vi "HFRR ADV v018 new software.vi"() -> ()   [LabVIEW 2025] (continued)
              }
            }
          }
        }
        n4002 = disable-structure shown="Disabled" {
          disable-tunnel: w4768 -> [w4777 _]
          disable-tunnel: [w4776 _] -> w4767
          frame Disabled {
            n4003 = local read "Json St Flg"() -> (w4775:bool)
            n4004 = case shown="True" w4775 {
              tunnel: w4777 -> [w4778 w4780]
              tunnel: [w4778 w4779] -> w4776
              frame False {
              }
              frame True {
                n4005 = Increment(x=w4780) -> (x+1=w4779:dbl)
                "T cycle" <- w4779
                n4006 = local write "Json St Flg"(FALSE ("Json St Flg")) -> ()
              }
            }
          }
          frame Enabled {
          }
        }
        n4007 = local read "Quit"() -> (w4762:bool)
      }
    }
    frame Enabled {
    }
  }
  n4008 = stacked-sequence {
    tunnel: [w5160] -> w40
    frame #0 {
      w5160 = FALSE ("Upload \nConfirmed")
      n4009 = local write "Upload \nConfirmed"(w5160) -> ()
      n4010 = local write "St Str"("") -> ()
    }
  }
  n4011 = disable-structure shown="Disabled" {
    disable-tunnel: w40 -> [w5161 _]
    frame Disabled {
      n4012 = case shown="True" {
        selector: _ -> [_ _]
        tunnel: w5161 -> [_ w5162]
        frame False {
        }
        frame True {
          n4013 = while {
            tunnel: [w5168] -> _
            tunnel: w5162 -> [_]
            i -> [w5168]
            stop <- w5163 stop-if-true
            n4014 = local read "Json End Flg"() -> (w5167:bool)
            n4015 = Wait (ms)(milliseconds to wait=u32 20 ("Refresh Rate (ms)")) -> ()  [unwired: 1 out]
            n4016 = local read "refresh flag"() -> (w5164:bool)
            n4017 = local read "RUN"() -> (w5165:bool)
            n4018 = And(x=w5165, y=w5164) -> (x .and. y?=w5166:bool)
            n4019 = Or(x=w5166, y=w5167) -> (x .or. y?=w5169:bool)
            "AR Led" <- w5169
            n4020 = case shown="True" w5169 {
              frame False {
              }
              frame True {
                w5186 = "\",\""
                n4021 = local read "UUID"() -> (w5184:string)
                n4022 = local write "refresh flag"(FALSE ("refresh flag")) -> ()
                n4023 = local read "time"() -> (w5173:dbl)
                n4024 = Multiply(x=w5173, y=60.0) -> (x*y=w5172:dbl)
                n4025 = Concatenate Strings("UUID\" : \"", w5184, "\"}") -> (w5187:string)
                n4026 = Number To Fractional String(number=w5172, width (-)=i16 10, precision (6)=i16 4) -> (F-format string=w5201:string)  [unwired: 1 in]
                n4027 = Concatenate Strings("{", "\"Time\":\"", w5201, w5186) -> (w5196:string)
                n4028 = stacked-sequence {
                  tunnel: w5186 -> [w5249 w5257 w5264 w5272 w5280 w5289 w5296]
                  tunnel: [w5250 _ _ _ _ _ _] -> w5200
                  tunnel: [_ w5258 _ _ _ _ _] -> w5199
                  tunnel: [_ _ w5265 _ _ _ _] -> w5198
                  tunnel: [_ _ _ w5274 _ _ _] -> w5197
                  tunnel: w5187 -> [_ _ _ _ _ _ w5307]
                  tunnel: [_ _ _ _ _ _ w5306] -> w5183
                  tunnel: [_ _ _ _ _ w5286 _] -> w5182
                  tunnel: [_ _ _ _ w5279 _ _] -> w5181
                  frame #0 {
                    n4029 = local read "NORMAL LOAD"() -> (w5248:dbl)
                    n4030 = Number To Fractional String(number=w5248, width (-)=i16 10, precision (6)=i16 4) -> (F-format string=w5251:string)  [unwired: 1 in]
                    n4031 = Concatenate Strings("NormalLoad\":\"", w5251, w5249) -> (w5250:string)
                  }
                  frame #1 {
                    n4032 = local read "Temp"() -> (w5256:dbl)
                    n4033 = Number To Fractional String(number=w5256, width (-)=i16 10, precision (6)=i16 4) -> (F-format string=w5259:string)  [unwired: 1 in]
                    n4034 = Concatenate Strings("Temperature\":\"", w5259, w5257) -> (w5258:string)
                  }
                  frame #2 {
                    n4035 = local read "cof"() -> (w5262:dbl)
                    n4036 = Number To Fractional String(number=w5262, width (-)=i16 10, precision (6)=i16 4) -> (F-format string=w5266:string)  [unwired: 1 in]
                    n4037 = Concatenate Strings("FrictionalForce\":\"", w5266, w5264) -> (w5265:string)
                  }
                  frame #3 {
                    n4038 = local read "Set Hz"() -> (w5270:dbl)
                    n4039 = Multiply(x=w5270, y=60.0) -> (x*y=w5269:dbl)
                    n4040 = Number To Fractional String(number=w5269, width (-)=i16 10, precision (6)=i16 4) -> (F-format string=w5275:string)  [unwired: 1 in]
                    n4041 = Concatenate Strings("Speed\":\"", w5275, w5272) -> (w5274:string)
                  }
                  frame #4 {
                    n4042 = local read item#-1() -> (w5278)
                    n4043 = Number To Fractional String(number=w5278, width (-)=i16 10, precision (6)=i16 4) -> (F-format string=w5282:string)  [unwired: 1 in]
                    n4044 = Concatenate Strings("LinearDeformation\":\"", w5282, w5280) -> (w5279:string)
                  }
                  frame #5 {
                    n4045 = local read "AIR TEMP"() -> (w5285:dbl)
                    n4046 = local read "Json St Flg"() -> (w5287:bool)
                    n4047 = local read "Json End Flg"() -> (w5288:bool)
                    n4048 = Number To Fractional String(number=w5285, width (-)=i16 10, precision (6)=i16 4) -> (F-format string=w5291:string)  [unwired: 1 in]
                    n4049 = Concatenate Strings("Vibration\":\"", w5291, w5289) -> (w5286:string)
                    n4050 = And(x=w5287, y=w5288) -> ()  [unwired: 1 out]
                  }
                  frame #6 {
                    n4051 = local read "Json End Flg"() -> (w5295:bool)
                    n4052 = Get Date/Time In Seconds() -> (seconds since 1Jan1904=w5303:timestamp)
                    n4053 = local read "Json St Flg"() -> (w5294:bool)
                    n4054 = To Double Precision Float(number=w5303) -> (double precision float=w5302:dbl)
                    n4055 = Subtract(x=w5302, y=2082844800.0) -> (x-y=w5300:dbl)
                    n4056 = Number To Fractional String(number=w5300, width (-)=i16 12, precision (6)=i16 0) -> (F-format string=w5297:string)  [unwired: 1 in]
                    n4057 = case shown="True" w5295 {
                      tunnel: ["" w5310] -> w5304
                      tunnel: w5297 -> [_ w5311]
                      tunnel: w5296 -> [_ w5309]
                      frame False {
                      }
                      frame True {
                        n4058 = local write "Json End Flg"(FALSE ("Json St Flg")) -> ()
                        n4059 = Concatenate Strings("End\": \"", w5311, w5309) -> (w5310:string)
                      }
                    }
                    n4060 = case shown="True" w5294 {
                      tunnel: [w5314 w5317] -> w5305
                      tunnel: w5297 -> [_ w5318]
                      tunnel: w5296 -> [_ w5315]
                      frame False {
                        n4061 = local read "St Str"() -> (w5314:string)
                      }
                      frame True {
                        n4062 = Concatenate Strings("Start\":\"", w5318, w5315) -> (w5317:string)
                        "St Str" <- w5317
                        n4063 = local write "Json St Flg"(FALSE ("Json St Flg")) -> ()
                      }
                    }
                    n4064 = Concatenate Strings(w5305, w5304, w5307) -> (w5306:string)
                  }
                }
                n4065 = local read "FILE"() -> (w5175:string)
                n4066 = Concatenate Strings("\",\"OperatorID\":\"" ("string"), "Operator ID") -> (w5178:string)
                n4067 = Concatenate Strings("\",\"DatasetTitle\":\"" ("string"), w5175) -> (w5177:string)
                n4068 = Concatenate Strings("\",\"SerialNumber\":\"" ("string"), "Serial No") -> (w5207:string)
                n4069 = Concatenate Strings("\",\"ModelNumber\":\"" ("string"), "Model No") -> (w5206:string)
                n4070 = Concatenate Strings(w5207, w5206) -> (w5189:string)
                n4071 = Concatenate Strings("{\"SecretKey\":\"", "Secret Key", w5189, w5178, w5177, "\",\"Samples\":[") -> (w5194:string)
                n4072 = Concatenate Strings(w5196, w5200, w5199, w5198, w5197, w5181, w5182, w5183) -> (w5195:string)
                n4073 = Concatenate Strings(w5194, w5195, "]}") -> (w5193:string)
                n4074 = stacked-sequence {
                  tunnel: w5193 -> [w5222 _ _]
                  tunnel: [_ _ w5239] -> _
                  frame #0 {
                    (unwired) FALSE ("convert eol (F)")
                    w5224 = enum16{"start", "end", "current"}."start" ("pos mode (0:2)")
                    n4075 = Path To String(path="Path") -> (string=w5230:string)
                    n4076 = Concatenate Strings(w5230, "\\", "Data File Name") -> (w5232:string)
                    n4077 = local write "standard output"(" ") -> ()
                    n4078 = String To Path(string=w5232) -> (path=w5221:path)
                    n4079 = call <vilib>:"Open_Create_Replace File.vi"("advisory dialog? (display:T)"=FALSE, "function (open:0)"=T32."create or replace", "file path"=w5221) -> ("error out"=w5235:errorcluster, "refnum"=w5234:refnum<file>)  [unwired: 5 in, 2 out]
                    n4080 = Set File Position(refnum=w5234, from (0:start)=w5224, error in=w5235) -> (refnum out=w5215:refnum<file>, error out=w5214:errorcluster)  [unwired: 1 in]
                    n4081 = Write to Binary File(file (use dialog)=w5215, data=" ", error in=w5214, 5:FALSE ("prepend array or string size? (T)")) -> (refnum out=w5225:refnum<file>, error out=w5226:errorcluster)  [unwired: 2 in, 1 out]
                    n4082 = Set File Position(offset (in bytes) (0)=w5224, refnum=w5225, error in=w5226) -> (refnum out=w5218:refnum<file>, error out=w5217:errorcluster)  [unwired: 1 in]
                    n4083 = Write to Binary File(file (use dialog)=w5218, data=w5222, error in=w5217, 5:FALSE ("prepend array or string size? (T)")) -> (error out=w5220:errorcluster)  [unwired: 2 in, 2 out]
                    n4084 = flat-sequence {
                      tunnel: w5221 -> [w5237]
                      tunnel: w5220 -> [_]
                      frame #0 {
                        n4085 = call <vilib>:"Read Characters From File.vi"("file path (dialog if empty)"=w5237) -> ("character string"=→"JSON string":string)  [unwired: 5 in, 3 out]
                      }
                    }
                    "SinglePoint" <- w5222
                  }
                  frame #1 {
                  }
                  frame #2 {
                    (unwired) "\"Stored\": true" ("string")
                    n4086 = call <vilib>:"System Exec.vi"("run minimized? (F)"=TRUE, "wait until completion? (T)"=TRUE, "working directory"=path "C:/LAB-IQ-NXT", "command line"="C:\\LAB-IQ-NXT\\JPost.bat") -> ("standard error"=→"Respose From Server":string, "standard output"=w5242:string)  [unwired: 4 in, 2 out]
                    "standard output" <- w5242
                    n4087 = Match Pattern(string=w5242, regular expression="JSON Check String") -> (match substring=w5240:string, offset past match=w5239:i32)  [unwired: 1 in, 2 out]
                    n4088 = Equal?(x=w5240, y="JSON Check String") -> (x = y?=→"Upload \nConfirmed":bool)
                  }
                }
              }
            }
            n4089 = local read "Quit"() -> (w5163:bool)
          }
        }
      }
    }
    frame Enabled {
    }
  }
  n4090 = disable-structure shown="Disabled" {
    disable-tunnel: _ -> [w5325 _]
    frame Disabled {
      n4091 = while {
        shift-right: [w5333] -> w5321
        shift-left: _ -> [w5334]
        shift-right: [w5331] -> w5322
        shift-left: errorcluster {"status"=TRUE, "code"=0, "source"="Init"} ("error out") -> [w5332]
        shift-right: [w5329] -> _
        shift-left: "" -> [w5330]
        tunnel: [w5327] -> _
        tunnel: w5325 -> [_]
        i -> [w5327]
        stop <- w5326 stop-if-true
        n4092 = flat-sequence {
          tunnel: [w5335] -> w5328
          frame #0 {
            n4093 = Wait (ms)(milliseconds to wait=10.0 ("Delay")) -> (millisecond timer value=w5335:u32)
          }
        }
        n4094 = case shown="No Error" w5332 {
          selector: w5332 -> [w5365 w5484]
          tunnel: [w5348 w5486] -> w5333
          tunnel: [w5347 w5485] -> w5331
          tunnel: w5334 -> [w5366 w5478]
          tunnel: w5330 -> [w5346 w5477]
          tunnel: [w5345 w5477] -> w5329
          tunnel: w5328 -> [_ _]
          frame No Error {
            n4095 = Concatenate Strings("\r", "\n") -> (w5357:string)  [unwired: 1 in]
            n4096 = case shown="True" w5358 {
              tunnel: w5366 -> [w5390 w5397]
              tunnel: w5365 -> [w5389 w5396]
              tunnel: [w5390 w5395] -> w5364
              tunnel: [w5389 w5394] -> w5344
              tunnel: w5357 -> [_ w5393]
              frame False {
              }
              frame True {
                n4097 = VISA Write(VISA resource name=w5397, write buffer=w5393, error in (no error)=w5396) -> (VISA resource name out=w5395:refnum<visa-resource-name>, error out=w5394:errorcluster)  [unwired: 1 out]
                n4098 = local write "Read String"("") -> ()
                n4099 = local write item#-1(FALSE) -> ()
              }
            }
            n4100 = property class="Instr"(reference=w5364, error in=w5344) -> (reference out=w5363:refnum<visa-resource-name>, error out=w5362:errorcluster, "Serial Settings:Number of Bytes at Serial Port"=w5361:u32)
            n4101 = Greater?(x=w5361, y=u32 100) -> (0:w5359:bool)
            n4102 = case shown="True" w5359 {
              tunnel: w5363 -> [w5400 w5424]
              tunnel: w5362 -> [w5399 w5423]
              tunnel: w5361 -> [_ w5422]
              tunnel: [w5400 w5421] -> w5350
              tunnel: [w5399 w5420] -> w5349
              tunnel: w5346 -> [w5398 w5419]
              tunnel: [w5398 ""] -> w5345
              frame False {
              }
              frame True {
                w5409 = u32 6 ("y")
                # "Page 84 of \nmanual"
                n4103 = VISA Read(VISA resource name=w5424, byte count=w5422, error in (no error)=w5423) -> (VISA resource name out=w5421:refnum<visa-resource-name>, read buffer=w5417:string, error out=w5420:errorcluster)  [unwired: 1 out]
                n4104 = while {
                  tunnel: w5417 -> [w5473]
                  tunnel: [w5469] -> w5411 mode=indexing
                  tunnel: [w5463] -> w5415 mode=indexing
                  tunnel: [w5461] -> _
                  i -> [w5461]
                  stop <- w5466 stop-if-true
                  n4105 = String Subset(string=w5473, offset (0)=w5461) -> (substring=w5468:string)  [unwired: 1 in]
                  n4106 = String To Byte Array(string=w5468) -> (unsigned byte array=w5472:u8[])
                  n4107 = String Length(string=w5468) -> (length=w5467:i32)
                  n4108 = Index Array(array=w5472) -> (element=w5471:u8)  [unwired: 1 in]
                  n4109 = Equal To 0?(x=w5467) -> (x = 0?=w5466:bool)
                  n4110 = Number To Boolean Array(number=w5471) -> (Boolean array=w5465:bool[])
                  n4111 = Reverse 1D Array(array=w5465) -> (reversed array=w5464:bool[])
                  n4112 = And(x=w5465, y=bool[] [FALSE, FALSE, FALSE, FALSE, FALSE, FALSE, TRUE, TRUE] ("Boolean array")) -> (x .and. y?=w5469:bool[])
                  n4113 = And(x=w5464, y=bool[] [FALSE, FALSE, TRUE, TRUE, TRUE, TRUE, TRUE, TRUE] ("Boolean array")) -> (x .and. y?=w5463:bool[])
                }
                n4114 = Concatenate Strings(w5419, w5417) -> (→"Read String":string)
                n4115 = while {
                  tunnel: w5411 -> [w5460] mode=indexing
                  tunnel: [w5456] -> w5414
                  i -> [w5456]
                  stop <- w5457 stop-if-true
                  n4116 = Search 1D Array(1D array=w5460, element=TRUE) -> (index of element=w5458:i32)  [unwired: 1 in]
                  n4117 = Less Than 0?(x=w5458) -> (x < 0?=w5457:bool)
                }
                n4118 = Delete From Array(array=w5415, length=w5414, index (row)=0) -> (array with subset deleted=w5410:bool[][])  [unwired: 1 in, 1 out]
                n4119 = Array Size(array=w5410) -> (size(s)=w5412:i32[])
                n4120 = Index Array(array=w5412) -> (element=w5404:i32)  [unwired: 1 in]
                n4121 = Greater?(x=w5404, y=w5409) -> (0:w5407:bool)
                n4122 = Subtract(x=w5404, y=w5409) -> (x-y=w5408:u32)
                n4123 = Select(t=w5408, s=w5407, f=u32 0) -> (s? t:f=w5405:u32)
                n4124 = while {
                  tunnel: w5410 -> [w5443]
                  tunnel: [w5445] -> w5403 mode=indexing
                  tunnel: w5405 -> [w5427]
                  i -> [w5444]
                  stop <- w5442 stop-if-true
                  w5434 = 6 ("index")
                  w5433 = 2 ("length")
                  # "Page 65 of \nmanual"
                  n4125 = Multiply(x=u32 3 ("y"), y=w5444) -> (x*y=w5441:u32)
                  n4126 = Divide(x=u32 102 ("y"), y=u32 65520) -> (x/y=w5451:dbl)
                  n4127 = Greater Or Equal?(x=w5441, y=w5427) -> (x >= y?=w5442:bool)
                  n4128 = Index Array(array=w5443, index (row) #1=w5441) -> (element #1=w5439:bool[], element #2=w5438:bool[], element #3=w5437:bool[])  [unwired: 5 in]
                  n4129 = Reverse 1D Array(array=w5439) -> (reversed array=w5432:bool[])
                  n4130 = Reverse 1D Array(array=w5438) -> (reversed array=w5436:bool[])
                  n4131 = Reverse 1D Array(array=w5437) -> (reversed array=w5435:bool[])
                  n4132 = Delete From Array(array=w5432, length=w5433, index=w5434) -> (array with subset deleted=w5428:bool[])  [unwired: 1 out]
                  n4133 = Delete From Array(array=w5436, length=w5433, index=w5434) -> (array with subset deleted=w5429:bool[])  [unwired: 1 out]
                  n4134 = Delete From Array(array=w5435, length=w5433, index=w5434) -> (array with subset deleted=w5430:bool[])  [unwired: 1 out]
                  n4135 = Insert Into Array(array=bool[] [] ("Boolean array"), new element #1=w5428, new element #2=w5429, new element #3=w5430) -> (w5431:bool[])  [unwired: 1 in]
                  n4136 = Boolean Array To Number(Boolean array=w5431) -> (number=w5440:u32)
                  n4137 = Multiply(x=w5451, y=w5440) -> (x*y=w5450:dbl)
                  n4138 = Decrement(x=w5450) -> (x-1=w5449:dbl)
                  n4139 = Divide(x=w5449, y=u32 100) -> (x/y=w5447:dbl)
                  n4140 = Multiply(x=w5447, y=u32 10) -> (x*y=w5445:dbl)
                }
                n4141 = Delete From Array(array=w5403) -> (array with subset deleted=w5402:dbl[])  [unwired: 2 in, 1 out]
                "Waveform Graph 5" <- w5402
                "Waveform Chart 3" <- w5402
                n4142 = call-poly <vilib>:"Mean.vi"("X"=w5402) -> ("mean"=w5401:dbl)  [unwired: 1 out]
                n4143 = case shown="True" {
                  selector: _ -> [_ _]
                  tunnel: w5401 -> [_ w5426]
                  frame False {
                  }
                  frame True {
                    n4144 = local write item#-1(FALSE ("Zero 4")) -> ()
                    "z_measure" <- w5426
                  }
                }
              }
            }
            n4145 = local read item#-1() -> (w5341)
            n4146 = local read item#-1() -> (w5340)
            n4147 = local read item#-1() -> (w5342)
            n4148 = local read item#-1() -> (w5339)
            n4149 = case shown="True" w5337 {
              tunnel: w5341 -> [_ w5369]
              tunnel: w5342 -> [_ w5368]
              frame False {
              }
              frame True {
                n4150 = Build Array(w5369, w5368) -> (w5367:void[])
                n4151 = local read item#-1() -> (w5372)
                n4152 = Build Array (concatenate)(w5372, w5367) -> (w5370:void[])
                n4153 = local write item#-1(w5370) -> ()
                n4154 = local write item#-1(FALSE ("Boolean 8")) -> ()
              }
            }
            n4155 = call "Build XY Graph"("Enable"=w5339, "Reset"=w5340, "Y Input"=w5342, "X Input"=w5341) -> ("XY Graph"=w5338:cluster{"Y":dbl[], "Y":dbl[]}[])  [unwired: 6 in, 1 out]
            n4156 = case shown="True" {
              selector: _ -> [_ _]
              frame False {
              }
              frame True {
                n4157 = local read item#-1() -> (w5373)
                n4158 = Index Array(array=w5373, index (col) #1=0 ("disabled index (col)"), index (col) #2=1 ("index (col)")) -> (element #1=w5375, element #2=w5374)  [unwired: 2 in]
                n4159 = call <vilib>:"Linear Fit.vi"("Y"=w5375, "X"=w5374) -> ()  [unwired: 9 in, 5 out]
                n4160 = local write item#-1(FALSE ("Boolean 9")) -> ()
              }
            }
            n4161 = case shown="True" {
              selector: _ -> [_ _]
              frame False {
              }
              frame True {
                n4162 = local write item#-1(dbl[][] [] ("Captured Values")) -> ()
                n4163 = local write item#-1(FALSE ("Boolean 7")) -> ()
              }
            }
            n4164 = Concatenate Strings("\r", "\n") -> (w5352:string, w5351:string)
            n4165 = case shown="True" w5343 {
              tunnel: w5350 -> [w5382 w5388]
              tunnel: w5349 -> [w5381 w5387]
              tunnel: [w5382 w5386] -> w5348
              tunnel: [w5381 w5385] -> w5347
              tunnel: w5352 -> [_ w5384]
              frame False {
              }
              frame True {
                n4166 = VISA Write(VISA resource name=w5388, write buffer=w5384, error in (no error)=w5387) -> (VISA resource name out=w5386:refnum<visa-resource-name>, error out=w5385:errorcluster)  [unwired: 1 out]
                n4167 = local write item#-1(FALSE ("WRITE")) -> ()
              }
            }
          }
          frame Error {
            w5476 = u16 10 items=["1.0"=10, "1.5"=15, "2.0"=20] ("stop bits (10: 1 bit)")
            n4168 = Wait (ms)(milliseconds to wait=u32 20) -> ()  [unwired: 1 out]
            n4169 = VISA Close(VISA resource name=w5478, error in (no error)=w5484) -> (error out=w5483:errorcluster)
            n4170 = call <vilib>:"Clear Errors.vi"("error in (no error)"=w5483) -> ("error out"=w5482:errorcluster)  [unwired: 5 in, 1 out]
            n4171 = call-poly "VISA Configure Serial Port"("timeout (10sec)"=u32 200, "Enable Termination\nChar (T)"=TRUE ("Enable Termination\nChar (T)"), "baud rate (9600)"=u32 921600, "error in (no error)"=w5482, "stop bits (10: 1 bit)"=w5476) -> ("VISA resource name"=w5474:refnum<visa-resource-name>, "VISA resource name out"=w5486:refnum<visa-resource-name>, "error out"=w5485:errorcluster)  [unwired: 8 in]
          }
        }
        n4172 = local read "Quit"() -> (w5326:bool)
      }
      n4173 = VISA Close(VISA resource name=w5321, error in (no error)=w5322) -> (error out=w5320:errorcluster)
      n4174 = call <vilib>:"Clear Errors.vi"("error in (no error)"=w5320) -> ()  [unwired: 5 in, 2 out]
    }
    frame Enabled {
    }
  }
  n4175 = disable-structure shown="Disabled" {
    disable-tunnel: _ -> [w5491 _]
    frame Disabled {
      n4176 = while {
        tunnel: [w5498] -> _
        shift-right: [w5495] -> w5488
        shift-left: _ -> [w5497]
        shift-right: [w5496] -> w5489
        shift-left: errorcluster {"status"=TRUE, "code"=0, "source"="Init"} ("error out") -> [w5494]
        tunnel: w5491 -> [_]
        i -> [w5498]
        stop <- w5492 stop-if-true
        n4177 = flat-sequence {
          tunnel: w5494 -> [w5589]
          tunnel: [w5589] -> w5493
          frame #0 {
            n4178 = Wait (ms)(milliseconds to wait=u32 50) -> ()  [unwired: 1 out]
          }
        }
        n4179 = case shown="No Error" w5493 {
          selector: w5493 -> [w5539 w5582]
          tunnel: w5497 -> [w5538 w5581]
          tunnel: [w5505 w5572] -> w5496
          tunnel: [w5506 w5580] -> w5495
          frame No Error {
            w5532 = T33 {"Mode"=enum."RTU", "Slave Address"=1} ("Serial Parameters")
            n4180 = call-poly <vilib>:"MB Serial Master Query (poly).vi"("VISA resource name"=w5538, "Starting Address"=i16 1000, "Quantity"=u16 1, "Timeout"=u32 1000, "error in"=w5539, "Serial Parameters"=w5532) -> ("VISA resource name out"=w5533:refnum<visa-resource-name>, "Input Registers"=w5535:u16[], "error out"=w5531:errorcluster)  [unwired: 10 in, 1 out]
            n4181 = Random Number (0-1)() -> (number: 0 to 1=w5520:dbl)
            n4182 = Index Array(array=w5535, index=0) -> (element=w5530:u16)
            n4183 = Subtract(x=w5520, y=0.5) -> (x-y=w5519:dbl)
            n4184 = Divide(x=w5530, y=10 ("index")) -> (x/y=w5524:dbl)
            n4185 = Multiply(x=w5519, y=0.5) -> (x*y=w5518:dbl)
            n4186 = Add(x=w5524, y=w5518) -> (x+y=w5523:dbl)
            n4187 = local read "Amb temp"() -> (w5507:dbl)
            n4188 = Multiply(x=w5523, y=0.2) -> (x*y=w5527:dbl)
            n4189 = Multiply(x=w5507, y=0.8) -> (x*y=w5525:dbl)
            n4190 = Add(x=w5527, y=w5525) -> (x+y=w5508:dbl)
            n4191 = local read "set temp old"() -> (w5502:dbl)
            n4192 = local write "Amb temp"(w5508) -> ()
            n4193 = Select(t="SetTemp 2", s="Heater", f=100.0) -> (s? t:f=w5503:dbl)
            n4194 = Not Equal?(x=w5503, y=w5502) -> (x != y?=w5501:bool)
            n4195 = case shown="True" w5501 {
              tunnel: w5533 -> [w5567 w5569]
              tunnel: [w5566 w5569] -> w5513
              tunnel: w5531 -> [w5565 w5568]
              tunnel: [w5564 w5568] -> w5511
              tunnel: w5503 -> [w5559 _]
              tunnel: w5532 -> [w5561 w5570]
              tunnel: [w5561 w5570] -> w5514
              frame True {
                n4196 = Multiply(x=w5559, y=10 ("index")) -> (x*y=w5558:dbl)
                n4197 = call-poly <vilib>:"MB Serial Master Query (poly).vi"("VISA resource name"=w5567, "Address"=u16 0, "Holding Register"=w5558, "Timeout"=u32 1000, "error in"=w5565, "Serial Parameters"=w5561) -> ("VISA resource name out"=w5566:refnum<visa-resource-name>, "error out"=w5564:errorcluster)  [unwired: 11 in, 1 out]
                "set temp old" <- w5559
              }
              frame False {
              }
            }
            n4198 = flat-sequence {
              tunnel: [w5540] -> _
              tunnel: [w5540] -> w5510
              tunnel: w5511 -> [w5540]
              frame #0 {
                n4199 = Wait (ms)(milliseconds to wait=u32 100) -> ()  [unwired: 1 out]
              }
            }
            n4200 = call "Elapsed Time12"("Time Target (s)"=2.0, "Auto Reset"=TRUE) -> ("Time has Elapsed"=w5515:bool)  [unwired: 10 in, 7 out]
            n4201 = case shown="True" w5515 {
              tunnel: w5514 -> [w5544 w5557]
              tunnel: [w5544 w5557] -> _
              tunnel: [w5543 w5555] -> w5506
              tunnel: w5513 -> [w5543 w5556]
              tunnel: [w5542 w5553] -> w5505
              tunnel: w5510 -> [w5542 w5554]
              frame False {
              }
              frame True {
                n4202 = call-poly <vilib>:"MB Serial Master Query (poly).vi"("VISA resource name"=w5556, "Starting Address"=i16 1003 ("Addr"), "Quantity"=u16 1, "Timeout"=u32 1000, "error in"=w5554, "Serial Parameters"=w5557) -> ("VISA resource name out"=w5555:refnum<visa-resource-name>, "Input Registers"=w5550:u16[], "error out"=w5553:errorcluster)  [unwired: 10 in, 1 out]
                n4203 = Index Array(array=w5550, index=0) -> (element=w5549:u16)
                n4204 = Divide(x=w5549, y=u16 10) -> (x/y=w5545:dbl)
                n4205 = local write "set temp old"(w5545) -> ()
                n4206 = local write "SetTemp"(w5545) -> ()
              }
            }
            "Error Code" <- w5505
            n4207 = Unbundle(w5505) -> ("status"=→"TK4 status":bool)  [unwired: 2 out]
            "SetTemp" <- "SetTemp 2"
          }
          frame Error {
            w5584 = u16 0 items=["None", "Odd", "Even", "Mark", "Space"] ("Parity")
            w5585 = u16 0 items=["None", "XON/XOFF", "RTS/CTS", "XON/XOFF & RTS/CTS", "DTR/DSR", "XON/XOFF & DTR/DSR"] ("Flow Control")
            n4208 = VISA Clear(VISA resource name=w5581, error in (no error)=w5582) -> (VISA resource name out=w5575:refnum<visa-resource-name>, error out=w5573:errorcluster)
            n4209 = VISA Close(VISA resource name=w5575, error in (no error)=w5573) -> (error out=w5574:errorcluster)
            n4210 = call <vilib>:"Clear Errors.vi"("error in (no error)"=w5574) -> ("error out"=w5583:errorcluster)  [unwired: 5 in, 1 out]
            n4211 = Unbundle By Name(T33 {"Mode"=enum."RTU", "Slave Address"=1} ("input cluster")) -> ("Mode"=w5586:enum16{"RTU", "ASCII"})
            n4212 = call <vilib>:"MB Serial Init.vi"("Timeout"=u32 100, "Flow Control"=w5585, "Mode"=w5586, "error in (no error)"=w5583, "Parity"=w5584, "Baud Rate"=u32 9600, "VISA resource name"="Lubrication System COM Port :") -> ("error out"=w5572:errorcluster, "VISA resource name out"=w5580:refnum<visa-resource-name>)  [unwired: 3 in]
            n4213 = local write "set temp old"(0.0 ("set temp old")) -> ()
            n4214 = Unbundle(w5572) -> ("status"=w5571:bool)  [unwired: 2 out]
            n4215 = case shown="True" w5571 {
              selector: w5571 -> [_ w5588]
              frame False {
              }
              frame True {
                n4216 = local write "TK4 status"(w5588) -> ()
              }
            }
          }
        }
        n4217 = local read "Quit"() -> (w5492:bool)
      }
      n4218 = VISA Close(VISA resource name=w5488, error in (no error)=w5489) -> (error out=w5487:errorcluster)
      n4219 = call <vilib>:"Clear Errors.vi"("error in (no error)"=w5487) -> ()  [unwired: 5 in, 2 out]
    }
    frame Enabled {
    }
  }
